vi "EnvMillikReadChannel.vi"(8 "error in (no error)":errorcluster, 9 "timeout":i32, 10 "channel":string, 11 "VISA Refnum in":refnum<visa-resource-name>) -> (0 "error out":errorcluster, 1 "timestamp":string, 2 "read buffer":string, 3 "VISA Refnum out":refnum<visa-resource-name>, 5 "value":dbl)   [LabVIEW 2016]
uses:
  <vilib>/Instr/_visa.llb/Select Event Type.ctl
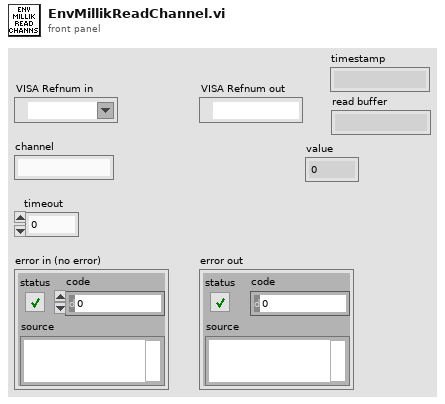
[diagram p1: front panel]
types:
  T1 = typedef "Select Event Type.ctl" = u32
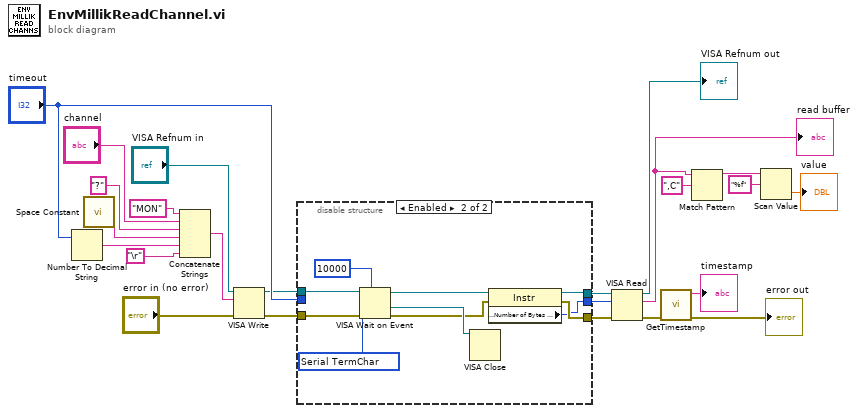
[diagram p0: block diagram]
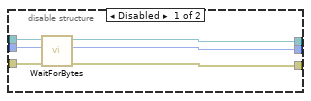
[diagram p2: hidden frame]
diagram:
  n1 = Number To Decimal String(number="timeout") -> (decimal integer string=w24:string)  [unwired: 1 in]
  n2 = call <vilib>:"Space Constant.vi"() -> ("String"=w12:string)
  n3 = Concatenate Strings("MON" ("write buffer"), "channel", "?" ("string"), w12, w24, "\r") -> (w14:string)
  n4 = VISA Write(VISA resource name="VISA Refnum in", write buffer=w14, error in (no error)="error in (no error)") -> (VISA resource name out=w18:refnum<visa-resource-name>, error out=w19:errorcluster)  [unwired: 1 out]
  n5 = disable-structure shown="Enabled" {
    disable-tunnel: "timeout" -> [w30 _]
    disable-tunnel: [w29 w34] -> w22
    disable-tunnel: [w28 w33] -> w21
    disable-tunnel: [w27 w35] -> w20
    disable-tunnel: w19 -> [w26 w38]
    disable-tunnel: w18 -> [w25 w40]
    frame Disabled {
      n6 = call "WaitForBytes.vi"("error in (no error)"=w26, "timeout [s]"=w30, "VISA Refnum in"=w25) -> ("error out"=w29:errorcluster, "Bytes at Port"=w28:u32, "VISA Refnum out"=w27:refnum<visa-resource-name>)  [unwired: 6 in]
    }
    frame Enabled {
      w37 = T1 1073684516 items=["Service Request"=1073684491, "Trigger"=3221168138, "Clear"=1073684493, "VXI Signal"=1073684512, "VXI/VME Interrupt"=3221168161, "VXI/VME Sysfail"=1073684509, "VXI/VME Sysreset"=1073684510, "GPIB CIC"=1073684498, "GPIB Talk"=1073684499, "GPIB Listen"=1073684500, "PXI Interrupt"=1073684514, "Serial Break"=1073684515, "Serial TermChar"=1073684516, "Serial CTS"=1073684521, "Serial DSR"=1073684522, "Serial DCD"=1073684524, "Serial RI"=1073684526, "Serial Character"=1073684533, "USB Interrupt"=1073684535, "All Enabled"=1073709055] ("Event Type")
      n7 = VISA Wait on Event(7:u32 10000 ("timeout (0)"), 8:w38, 10:w37, 11:w40) -> (0:w32:errorcluster, 1:w36:refnum<visa-resource-name>, 3:w31:refnum<visa-resource-name>)  [unwired: 1 in, 1 out]
      n8 = VISA Close(VISA resource name=w36) -> ()  [unwired: 1 in, 1 out]
      n9 = property class="Instr"(reference=w31, error in=w32) -> (reference out=w35:refnum<visa-resource-name>, error out=w34:errorcluster, "Serial Settings:Number of Bytes at Serial Port"=w33:u32)
    }
  }
  n10 = VISA Read(VISA resource name=w20, byte count=w21, error in (no error)=w22) -> (VISA resource name out=→"VISA Refnum out":refnum<visa-resource-name>, read buffer=w1:string, error out=w8:errorcluster)  [unwired: 1 out]
  "read buffer" <- w1
  n11 = call "GetTimestamp.vi"("error in (no error)"=w8) -> ("error out"=→"error out":errorcluster, "date/time string"=→"timestamp":string)  [unwired: 9 in]
  n12 = Match Pattern(string=w1, regular expression=",C") -> (before substring=w2:string)  [unwired: 1 in, 3 out]
  n13 = Scan Value(string=w2, format string="%f") -> (value=→"value":dbl)  [unwired: 1 in, 1 out]
